vi "DRAFT7.vi"() -> ()   [LabVIEW 2021]
uses:
  <vilib>/Analysis/3filter.llb/Butterworth Filter (DBL).vi
  <vilib>/Analysis/NI_AALBase.lvlib
  <vilib>/ptbypt/NI_PtbyPt.lvlib
panel:
  out "Array Size 3":u32
  out "Waveform Graph 10":dynamicdata(graph)
  out "Waveform Graph 7":dynamicdata(graph)
  out "Array Size 2":u32
  out "Array Size":u32
  out "Elapsed time in ms":u32
  in  "stop":bool
  in  "error in (no error)":errorcluster
  out "error out":errorcluster
  in  "loop 1":i32
  out "Waveform Graph 6":dynamicdata(graph)
  out "Waveform Graph 5":dynamicdata(graph)
  out "Waveform Graph 4":dynamicdata(graph)
  out "Waveform Graph 3":dbl[](graph)
  out "Waveform Graph 2":dynamicdata(graph)
  in  "Boolean":bool
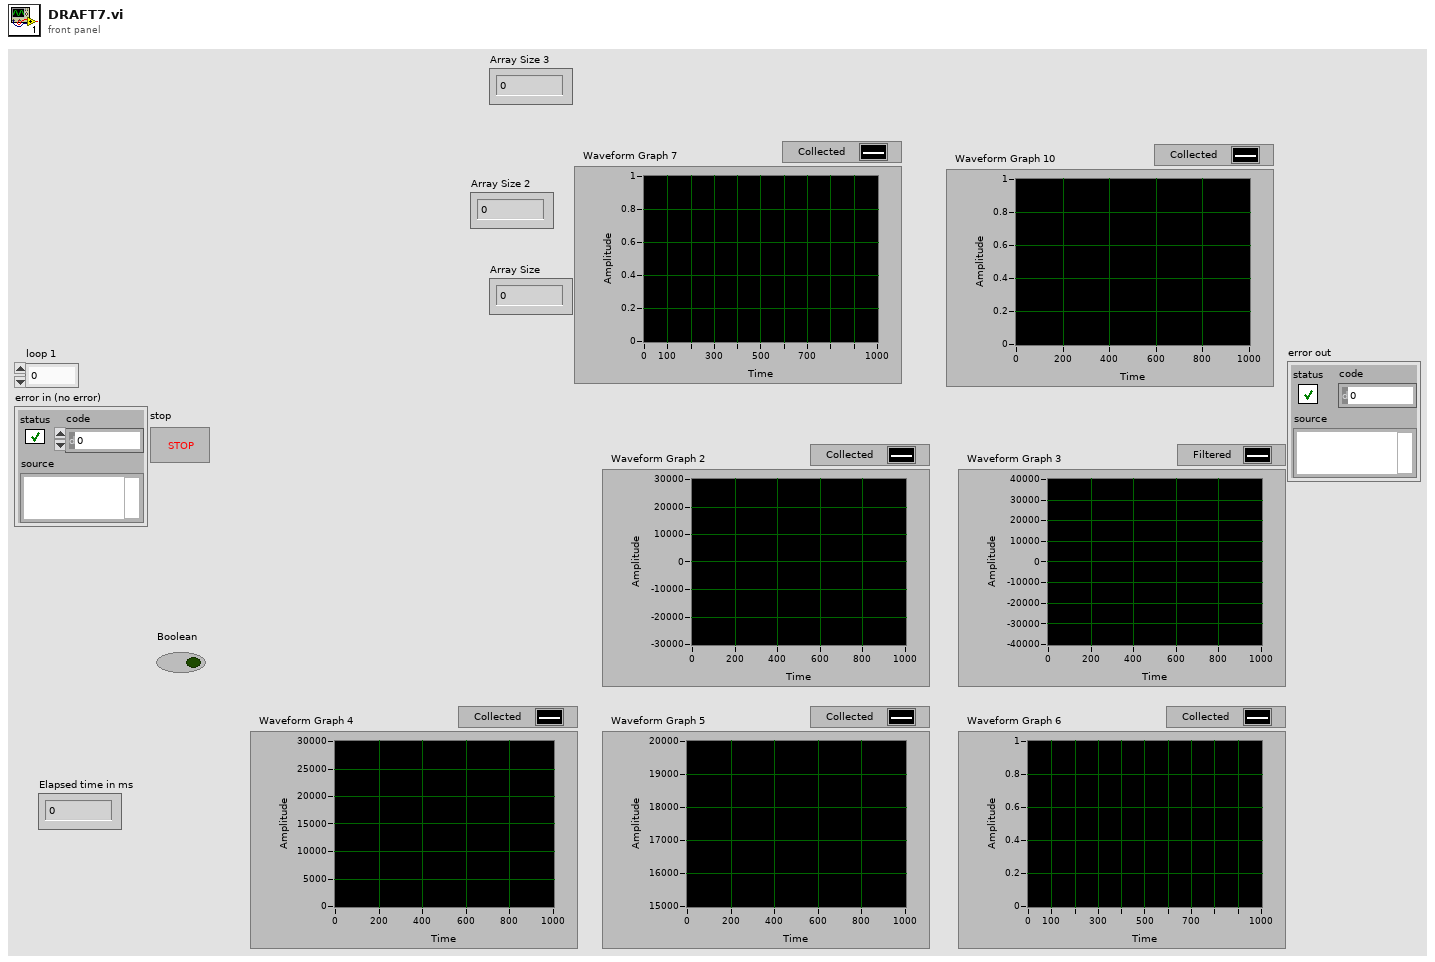
[diagram p1: front panel]
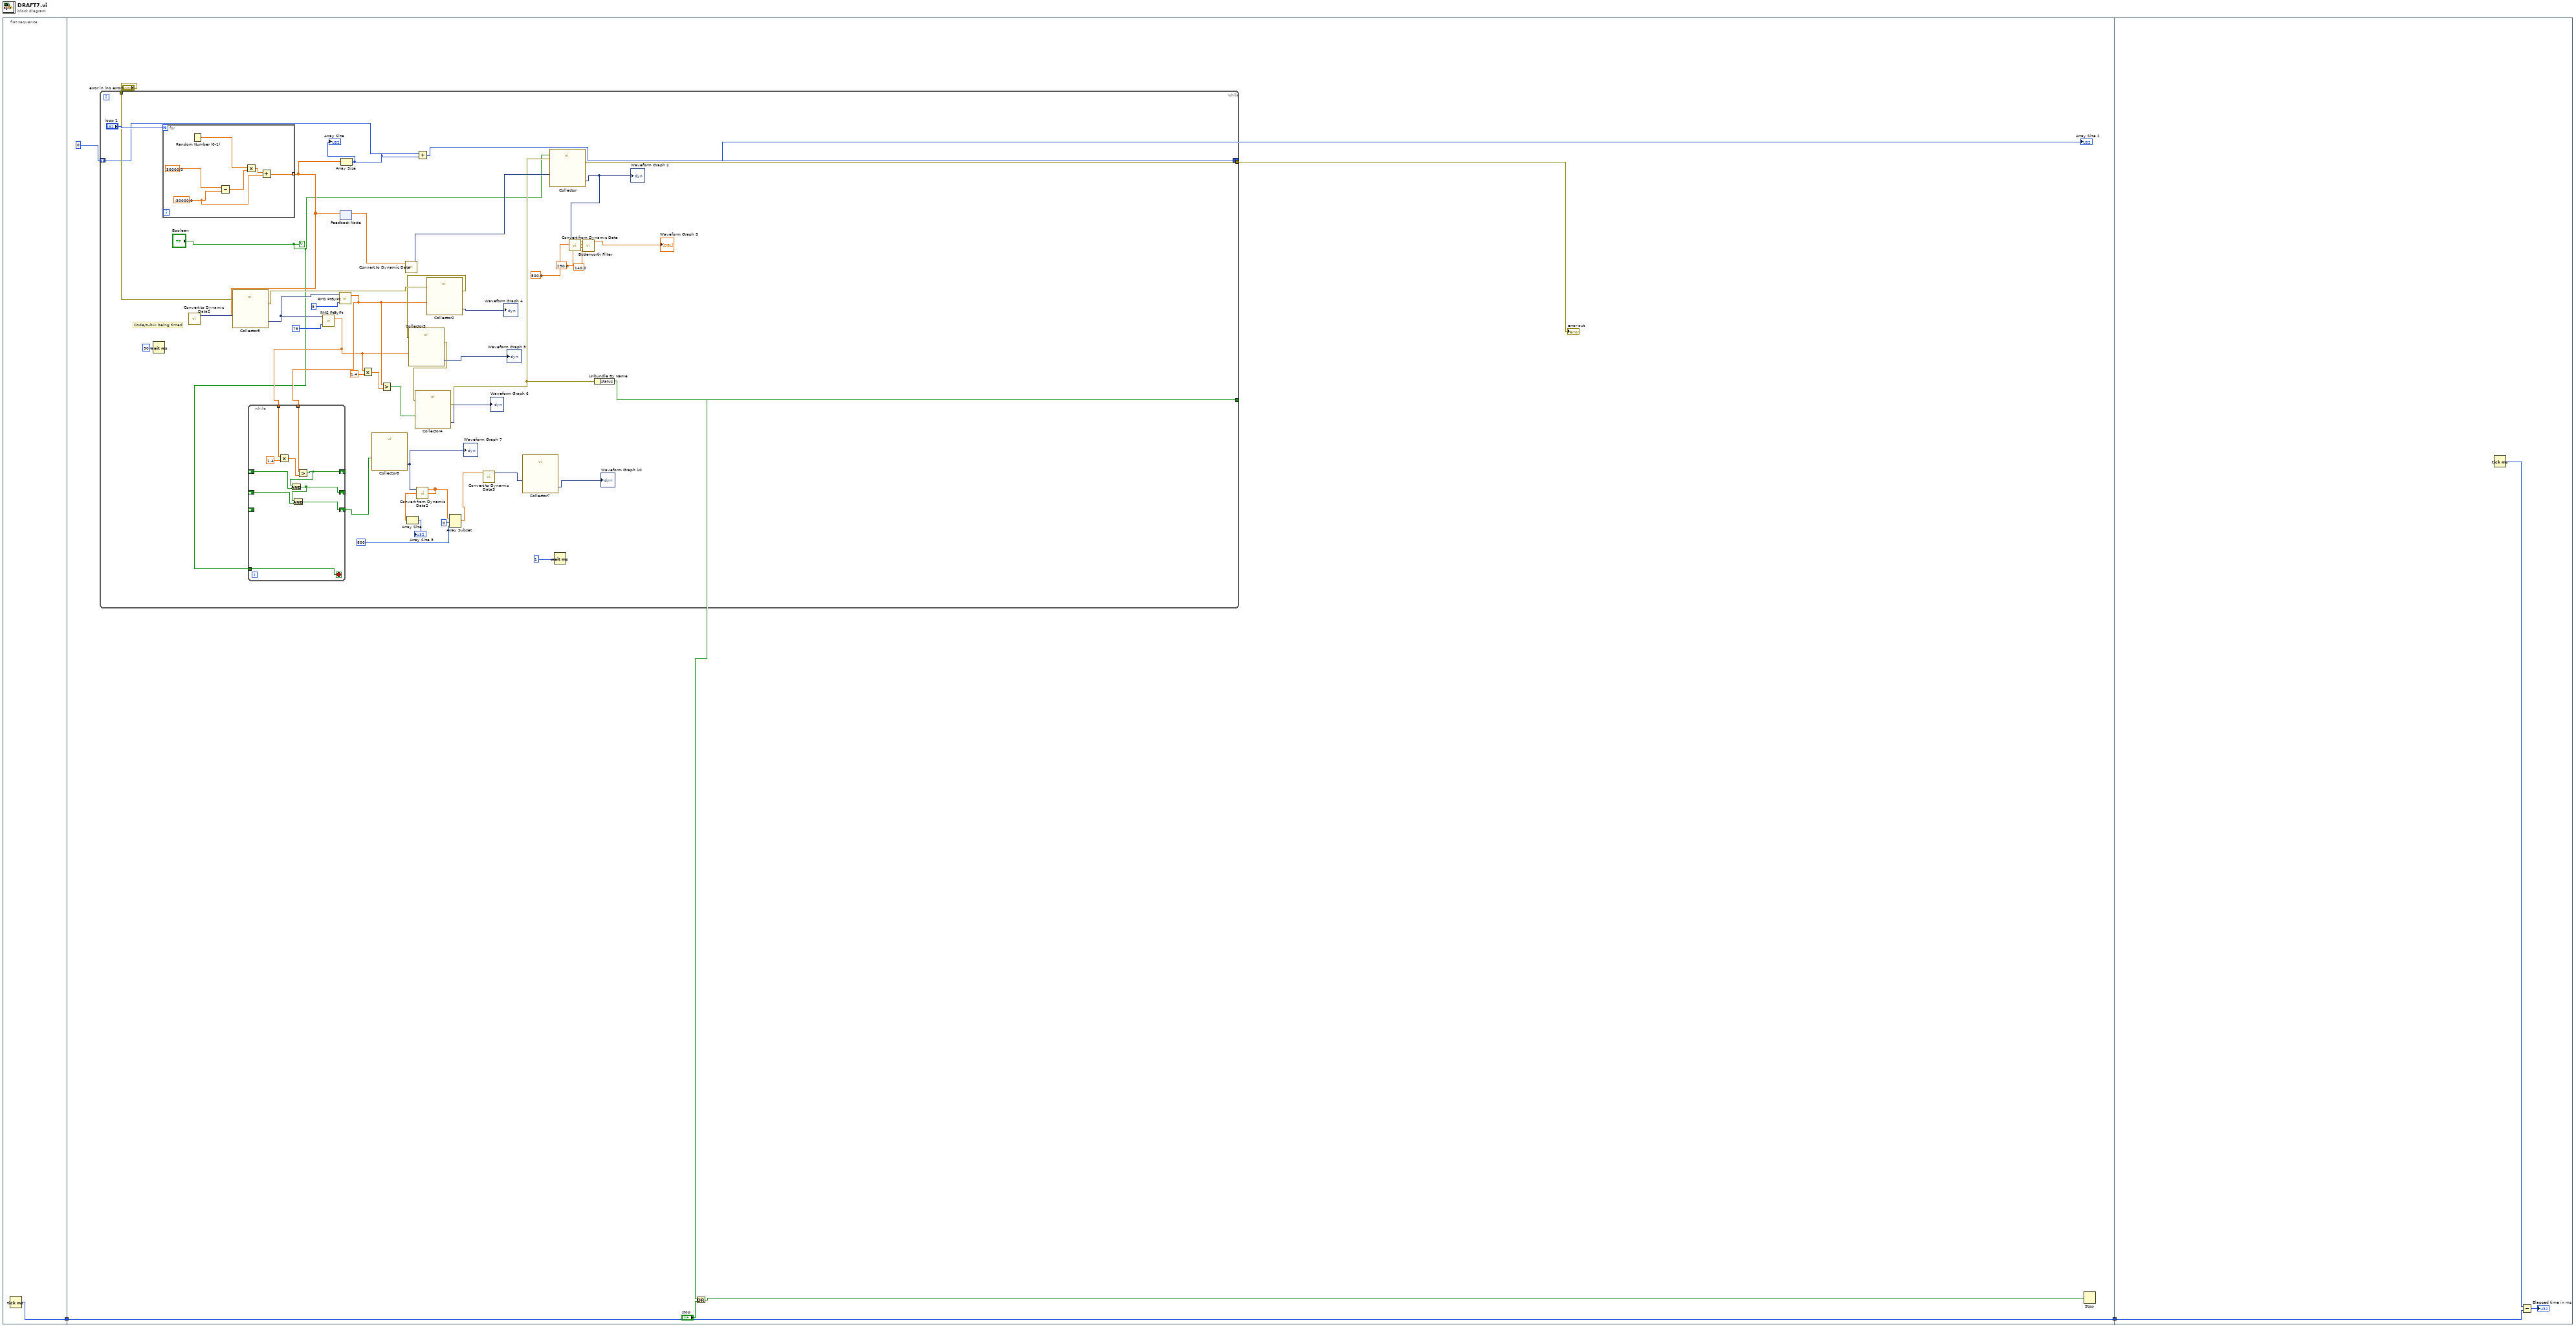
[diagram p0: block diagram]
diagram:
  n1 = flat-sequence {
    tunnel: [w3] -> w2
    tunnel: [w12] -> w1
    tunnel: w2 -> [w12]
    tunnel: w1 -> [w72]
    frame #0 {
      n2 = Tick Count (ms)() -> (millisecond timer value=w3:u32)
    }
    frame #1 {
      # "Code/subVI being timed"
      n3 = while {
        tunnel: "error in (no error)" -> [w37]
        tunnel: [w33] -> w9
        tunnel: [w31] -> w8
        shift-right: [w26] -> w4
        shift-left: 0 -> [w27]
        stop <- "Boolean" continue-if-true
        n4 = for {
          N: "loop 1" -> [_]
          tunnel: [w66] -> w29 mode=indexing
          w68 = -30000.0 ("y")
          n5 = Random Number (0-1)() -> (number: 0 to 1=w67:dbl)
          n6 = Subtract(x=30000.0, y=w68) -> (x-y=w71:dbl)
          n7 = Multiply(x=w67, y=w71) -> (x*y=w70:dbl)
          n8 = Add(x=w70, y=w68) -> (x+y=w66:dbl)
        }
        n9 = call "Convert to Dynamic Data2"("Array"=w29) -> ("Dynamic Data Type"=w39:dynamicdata)  [unwired: 3 in]
        n10 = call "Collector5"("error in (no error)"=w37, "Signals"=w39) -> ("error out"=w36:errorcluster, "Collected Signals"=w38:dynamicdata)  [unwired: 8 in]
        n11 = call <vilib>:"RMS PtByPt.vi"("sample length"=75, "x"=w38) -> ("rms value"=w24:dbl)  [unwired: 2 in, 1 out]
        n12 = call <vilib>:"RMS PtByPt.vi"("sample length"=3, "x"=w38) -> ("rms value"=w25:dbl)  [unwired: 2 in, 1 out]
        n13 = while {
          tunnel: w25 -> [w63]
          tunnel: w24 -> [w62]
          shift-right: [w57] -> _
          shift-left: _ -> [w58]
          shift-right: [w60] -> _
          shift-left: _ -> [w59]
          tunnel: "Boolean" -> [w61]
          shift-right: [w56] -> w21
          shift-left: _ -> [_]
          stop <- w61 stop-if-true
          n14 = Multiply(x=w62, y=1.4) -> (x*y=w64:dbl)
          n15 = Greater?(x=w63, y=w64) -> (0:w60:bool)
          n16 = And(x=w60, y=w59) -> (x .and. y?=w57:bool)
          n17 = And(x=w57, y=w58) -> (x .and. y?=w56:bool)
        }
        n18 = feedback-in #1(w29) -> ()
        n19 = feedback #1() -> (w30:dbl[])  [unwired: 1 in]
        n20 = Array Size(array=w29) -> (size(s)=w28:i32)
        "Array Size" <- w28
        n21 = Multiply(x=w24, y=1.4) -> (x*y=w43:dbl)
        n22 = call "Collector8"("Signals"=w21) -> ("Collected Signals"=w19:dynamicdata)  [unwired: 9 in, 1 out]
        "Waveform Graph 7" <- w19
        n23 = Greater?(x=w25, y=w43) -> (0:w42:bool)
        n24 = call "Convert to Dynamic Data"("Array"=w30) -> ("Dynamic Data Type"=w47:dynamicdata)  [unwired: 3 in]
        n25 = call "Convert from Dynamic Data2"("Dynamic Data Type"=w19) -> ("Array"=w16:dbl[])  [unwired: 3 in]
        n26 = Array Size(array=w16) -> (size(s)=→"Array Size 3":i32)
        n27 = Add(x=w28, y=w27) -> (x+y=w26:i32)
        n28 = call "Collector2"("error in (no error)"=w36, "Signals"=w25) -> ("error out"=w35:errorcluster, "Collected Signals"=→"Waveform Graph 4":dynamicdata)  [unwired: 8 in]
        n29 = call "Collector3"("error in (no error)"=w35, "Signals"=w24) -> ("error out"=w34:errorcluster, "Collected Signals"=→"Waveform Graph 5":dynamicdata)  [unwired: 8 in]
        n30 = call "Collector4"("error in (no error)"=w34, "Signals"=w42) -> ("error out"=w32:errorcluster, "Collected Signals"=→"Waveform Graph 6":dynamicdata)  [unwired: 8 in]
        n31 = Array Subset(array=w16, index=0, length=800 ("index")) -> (w14:dbl[])
        n32 = call "Convert to Dynamic Data3"("Array"=w14) -> ("Dynamic Data Type"=w20:dynamicdata)  [unwired: 3 in]
        n33 = call "Collector7"("Signals"=w20) -> ("Collected Signals"=→"Waveform Graph 10":dynamicdata)  [unwired: 9 in, 1 out]
        n34 = call "Collector"("error in (no error)"=w32, "Enable"="Boolean", "Signals"=w47) -> ("error out"=w33:errorcluster, "Collected Signals"=w50:dynamicdata)  [unwired: 7 in]
        "Waveform Graph 2" <- w50
        n35 = Wait (ms)(milliseconds to wait=u32 1 ("millisecond timer value")) -> ()  [unwired: 1 out]
        n36 = call "Convert from Dynamic Data"("Dynamic Data Type"=w50) -> ("Array"=w52:dbl[])  [unwired: 3 in]
        n37 = call-poly <vilib>:"Butterworth Filter.vi"("low cutoff freq: fl"=140.0, "high cutoff freq: fh"=250.0, "sampling freq: fs"=500.0, "X"=w52) -> ("Filtered X"=→"Waveform Graph 3":dbl[])  [unwired: 4 in, 1 out]
        n38 = Unbundle By Name(w32) -> ("status"=w31:bool)
      }
      "error out" <- w9
      "Array Size 2" <- w4
      n39 = Wait (ms)(milliseconds to wait=u32 50) -> ()  [unwired: 1 out]
      n40 = Or(x=w8, y="stop") -> (x .or. y?=w6:bool)
      n41 = Stop(stop? (T)=w6) -> ()
    }
    frame #2 {
      n42 = Tick Count (ms)() -> (millisecond timer value=w74:u32)
      n43 = Subtract(x=w74, y=w72) -> (x-y=→"Elapsed time in ms":u32)
    }
  }
